vi "Save File Parse File Name.vi"(0 "File String Name":path, 1 "Number of Cycles/ File":i32=1, 5 "Error In":errorcluster, 6 "Initialize.Washer In":T1={"Appliance Details"={"FileVersionInfo"={"FileVersion"="", "ProductName"="", "InternalName"="", "CompanyName"="", "LegalCopyright"="", "FileDescription"=""}, "Dishwasher Info"={"Open Cup Weight (gm):"=0.0, "Auto Cup Weight (gm):"=0.0, "Detergent-Dish:"="", "Inlet Temperature-Dish:"="", "Cycle Mode-Dish:"="", "Unit Control-Dish:"="", "Manufacturer-Dish:"=""}, "Washer Info"={"Hot Water Temperature (Fahrenheit):"="", "Cold Water Temperature (Fahrenheit):"="", "Capacity (cu.ft):"=0.0, "Initial Cloth Weight:"=0.0, "Cloth Lot:"=0, "Model Family:"="", "Program Name:"="", "Cycle Selection:"="", "Wash Temperature:"="", "Rinse Temperature:"="", "Load Size:"=""}, "File Name Output Array"=[], "Calibration Output Array"=[], "Appliance Common"={"Engineer:"="", "Model Number:"="", "Serial Number:"="", "Comments:"="", "Station ID:"="", "Technician:"="", "TR Number:"="", "Lab ID:"="", "Voltage:"="", "Water Pressure (PSI):"="", "Test Date:"="", "Computer Name:"="", "IP Address:"="", "Ambient RH:"="", "Frequency:"="", "Build:"="", "Filename:"="", "Test Type:"="", "Load Run #:"=0, "Ambient Temperature (F):"="", "File Path:"=path "", "Cycles Per Year"=60}, "Water Heater"={"Heating Mode:"=""}, "Dryer"={"Heat Setting:"="", "Washer Water Temperature (60 ± 5°F):"=60, "Water Hardness (PPM):"=17, "Dryness Setting:"="", "Dryer Type:"="", "Exhaust:"="", "Drying Cycle:"="", "Load Type:"="", "Nominal Load Weight"="", "Dryer Initial IMC Data"={"Measured IMC (lbs)"=7.0, "Actual Initial RMC (%)"=7.0, "RMC (Desired %)"=100.0, "Bone Dry Wt(lbs)"=7.0, "Tolerance(%)"=5.0, "Actual Final RMC (%)"=0.0, "CEF (lbf/kWh)"=0.0, "Minimum Weight (lbf)"=0.0, "Average Weight (lbf)"=0.0, "Maximum Weight (lbf)"=0.0, "Measured IMC In Range?"=FALSE, "Moisture Reduction Factor"=55.5, "Field Use Factor"=1.04, "Empty Dryer Cold Weigth"=0.0, "Energy Standard"=enum."D2-Automatic Dryer", "Weight Cloth (lbs)"=0.0, "Relative Moisture Content (%)"=0.0, "Relative Moisture Content - Avg (%)"=0.0}}}, "Display Data (RLT)"={"Status Color"=0, "Serial Number Display"="", "Cycle Count Display"=0, "Station Label Display"="", "Current Run Start Time Display"=0.0, "Board ID Display"="", "RPM Display"=0, "Current Display"=0.0, "Current Path Display"=path "", "Saving Display"=FALSE, "Unit Type Display"=enum."", "Total Time On Display"=0.0, "UI Button"=FALSE}} {"Display Data (RLT)"."Current Display" format="%.2f"; "Display Data (RLT)"."Cycle Count Display" format="%04d"; "Appliance Details"."Dryer"."Dryer Initial IMC Data"."Maximum Weight (lbf)" format="%03_6g"; "Appliance Details"."Dryer"."Dryer Initial IMC Data"."Average Weight (lbf)" format="%03_6g"; "Appliance Details"."Dryer"."Dryer Initial IMC Data"."Minimum Weight (lbf)" format="%03_6g"; "Appliance Details"."Dryer"."Dryer Initial IMC Data"."CEF (lbf/kWh)" format="%03_6g"; "Appliance Details"."Dryer"."Dryer Initial IMC Data"."Actual Final RMC (%)" format="%03_6g"; "Appliance Details"."Dryer"."Dryer Initial IMC Data"."Tolerance(%)" format="%0#_6g"; "Appliance Details"."Dryer"."Dryer Initial IMC Data"."Bone Dry Wt(lbs)" format="%03_6g"; "Appliance Details"."Dryer"."Dryer Initial IMC Data"."RMC (Desired %)" format="%0#_6g"; "Appliance Details"."Dryer"."Dryer Initial IMC Data"."Actual Initial RMC (%)" format="%03_6g"; "Appliance Details"."Dryer"."Dryer Initial IMC Data"."Measured IMC (lbs)" format="%0#_6g"}) -> (14 "Root Change?":bool, 15 "New File?":bool, 19 "Error Out":errorcluster)   [LabVIEW 2023, in "Save File.lvlib"]
uses:
  Save File.lvlib
  Public/Type Definitions/Save File Washer.ctl
  File Setup (Public)/Type Definition/Save File DISH Dishwasher Details.ctl
  <vilib>/Platform/fileVersionInfo.llb/FileVersionInformation.ctl
  Washer DOE/Type Definitions/DOE Appliance Common.ctl
  Custom Pallet Controls/Custom Pallet String.ctl
  File Setup (Public)/Type Definition/DPT IMC Data.ctl
  Washer DOE/Type Definitions/DOE Dryer Standard.ctl
  Public/Type Definitions/Save File Appliance Display.ctl
  Public/Type Definitions/Save File Unit Type.ctl
  File Setup.lvlib
panel:
  in  "Appliance Details.Appliance Common.TR Number:":string
  in  "Appliance Details.Appliance Common.Lab ID:":string
  in  "Appliance Details.Appliance Common.Serial Number:":string
  in  "Display Data (RLT).Cycle Count Display":i32
  in  "Debug":bool
  out "Save Array":bool[](array[boolean])
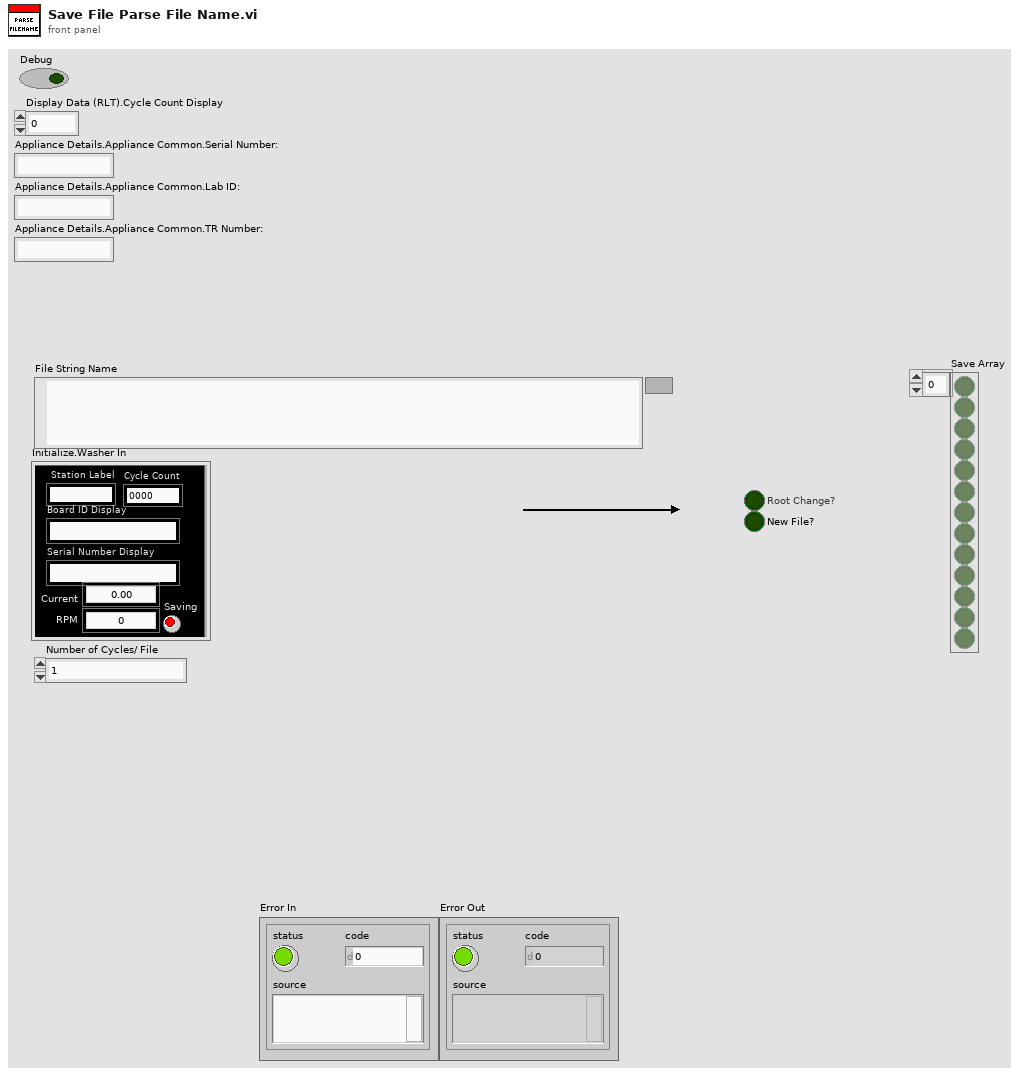
[diagram p1: front panel]
types:
  T1 = typedef "Save File.lvlib/Save File Washer.ctl" = cluster{"Appliance Details":T2, "Display Data (RLT)":T8}
  T2 = typedef "File Setup.lvlib/Save File DISH Dishwasher Details.ctl" = cluster{"FileVersionInfo":T3, "Dishwasher Info":cluster{"Open Cup Weight (gm):":dbl, "Auto Cup Weight (gm):":dbl, "Detergent-Dish:":string, "Inlet Temperature-Dish:":string, "Cycle Mode-Dish:":string, "Unit Control-Dish:":string, "Manufacturer-Dish:":string}, "Washer Info":cluster{"Hot Water Temperature (Fahrenheit):":string, "Cold Water Temperature (Fahrenheit):":string, "Capacity (cu.ft):":dbl, "Initial Cloth Weight:":dbl, "Cloth Lot:":i32, "Model Family:":string, "Program Name:":string, "Cycle Selection:":string, "Wash Temperature:":string, "Rinse Temperature:":string, "Load Size:":string}, "File Name Output Array":string[][], "Calibration Output Array":string[][], "Appliance Common":T4, "Water Heater":cluster{"Heating Mode:":string}, "Dryer":cluster{"Heat Setting:":T5, "Washer Water Temperature (60 ± 5°F):":u16, "Water Hardness (PPM):":u16, "Dryness Setting:":T5, "Dryer Type:":string, "Exhaust:":string, "Drying Cycle:":string, "Load Type:":string, "Nominal Load Weight":string, "Dryer Initial IMC Data":T6}}
  T3 = typedef "FileVersionInformation.ctl" = cluster{"FileVersion":string, "ProductName":string, "InternalName":string, "CompanyName":string, "LegalCopyright":string, "FileDescription":string}
  T4 = typedef "DOE Appliance Common.ctl" = cluster{"Engineer:":string, "Model Number:":string, "Serial Number:":string, "Comments:":string, "Station ID:":string, "Technician:":string, "TR Number:":string, "Lab ID:":string, "Voltage:":string, "Water Pressure (PSI):":string, "Test Date:":string, "Computer Name:":string, "IP Address:":string, "Ambient RH:":string, "Frequency:":string, "Build:":string, "Filename:":string, "Test Type:":string, "Load Run #:":i32, "Ambient Temperature (F):":string, "File Path:":path, "Cycles Per Year":u32}
  T5 = typedef "Custom Pallet String.ctl" = string
  T6 = typedef "DPT IMC Data.ctl" = cluster{"Measured IMC (lbs)":dbl, "Actual Initial RMC (%)":dbl, "RMC (Desired %)":dbl, "Bone Dry Wt(lbs)":dbl, "Tolerance(%)":dbl, "Actual Final RMC (%)":dbl, "CEF (lbf/kWh)":dbl, "Minimum Weight (lbf)":dbl, "Average Weight (lbf)":dbl, "Maximum Weight (lbf)":dbl, "Measured IMC In Range?":bool, "Moisture Reduction Factor":dbl, "Field Use Factor":dbl, "Empty Dryer Cold Weigth":dbl, "Energy Standard":T7, "Weight Cloth (lbs)":dbl, "Relative Moisture Content (%)":dbl, "Relative Moisture Content - Avg (%)":dbl}
  T7 = typedef "DOE Dryer Standard.ctl" = enum16{"D2-Automatic Dryer", "D2-Timer Dryer", "D1-Automatic Dryer", "D1-Timer Dryer", "Other"}
  T8 = typedef "Save File Appliance Display.ctl" = cluster{"Status Color":u32, "Serial Number Display":string, "Cycle Count Display":i32, "Station Label Display":string, "Current Run Start Time Display":dbl, "Board ID Display":string, "RPM Display":u32, "Current Display":dbl, "Current Path Display":path, "Saving Display":bool, "Unit Type Display":T9, "Total Time On Display":dbl, "UI Button":bool}
  T9 = typedef "Save File.lvlib/Save File Unit Type.ctl" = enum32{"", "Viper", "Hawk", "2015"}
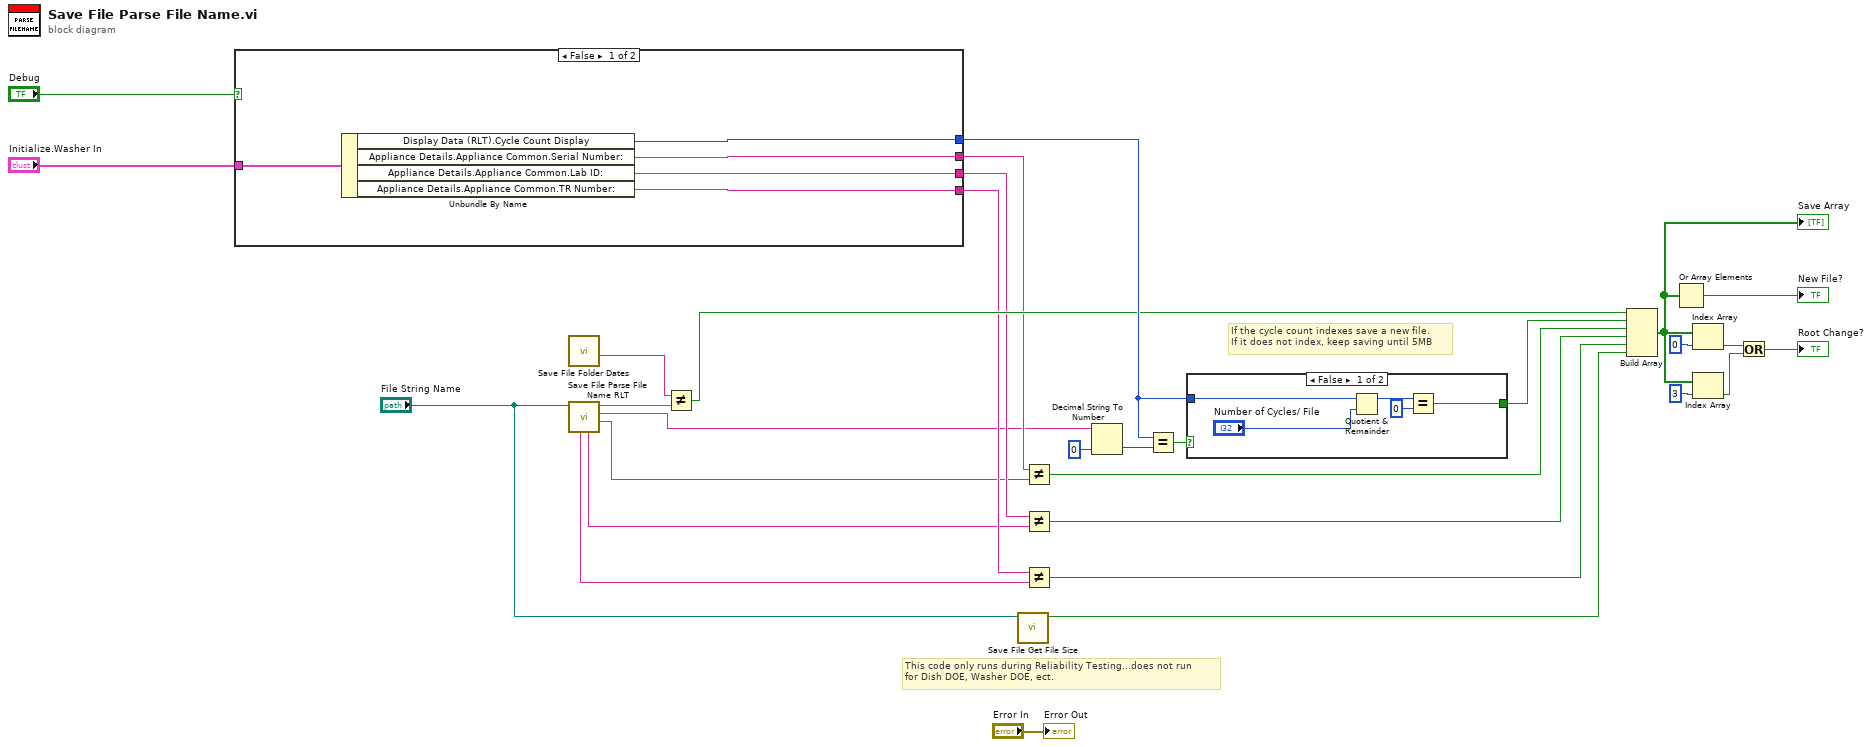
[diagram p0: block diagram]
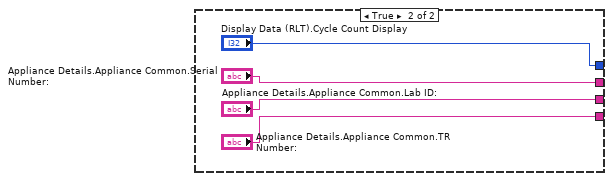
[diagram p2: hidden frame]
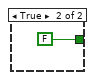
[diagram p3: hidden frame]
diagram:
  # "This code only runs during Reliability Testing...does not run \nfor Dish DOE, Washer DOE, ect."
  # "If the cycle count indexes save a new file.\nIf it does not index, keep saving until 5MB"
  n1 = case shown="False" "Debug" {
    tunnel: [w35 "Display Data (RLT).Cycle Count Display"] -> w27
    tunnel: "Initialize.Washer In" -> [w34 _]
    tunnel: [w33 "Appliance Details.Appliance Common.Serial Number:"] -> w11
    tunnel: [w32 "Appliance Details.Appliance Common.Lab ID:"] -> w10
    tunnel: [w31 "Appliance Details.Appliance Common.TR Number:"] -> w9
    frame False {
      n2 = Unbundle By Name(w34) -> ("Display Data (RLT).Cycle Count Display"=w35:i32, "Appliance Details.Appliance Common.Serial Number:"=w33:string, "Appliance Details.Appliance Common.Lab ID:"=w32:string, "Appliance Details.Appliance Common.TR Number:"=w31:string)
    }
    frame True {
    }
  }
  n3 = call "Save File Folder Dates.vi"() -> ("Year/Month/Day"=w28:string)  [unwired: 8 in, 3 out]
  n4 = call "Save File Parse File Name RLT.vi"("File String Name"="File String Name") -> ("Serial Number"=w3:string, "Cycle"=w4:string, "Date"=w7:string, "Lab ID"=w2:string, "TR Number"=w1:string)  [unwired: 5 in, 1 out]
  n5 = Not Equal?(x=w28, y=w7) -> (x != y?=w17:bool)
  n6 = call "Save File Get File Size.vi"("Old path"="File String Name") -> ("File Size Greater Than Limit"=w14:bool)  [unwired: 8 in, 2 out]
  n7 = Not Equal?(x=w11, y=w3) -> (x != y?=w13:bool)
  n8 = Not Equal?(x=w10, y=w2) -> (x != y?=w5:bool)
  n9 = Not Equal?(x=w9, y=w1) -> (x != y?=w12:bool)
  n10 = Decimal String To Number(string=w4, default (0L)=u16 0 ("default (0 I32)")) -> (number=w16:u16)  [unwired: 1 in, 1 out]
  n11 = Equal?(x=w27, y=w16) -> (x = y?=w25:bool)
  n12 = case shown="False" w25 {
    tunnel: w27 -> [w41 _]
    tunnel: [w40 FALSE] -> w26
    frame False {
      n13 = Quotient & Remainder(x=w41, y="Number of Cycles/ File") -> (x-y*floor(x/y)=w43:i32)  [unwired: 1 out]
      n14 = Equal?(x=w43, y=0) -> (x = y?=w40:bool)
    }
    frame True {
    }
  }
  n15 = Build Array(w17, w26, w13, w5, w12, w14) -> (w23:bool[])
  "Save Array" <- w23
  n16 = Or Array Elements(Boolean array=w23) -> (logical OR=→"New File?":bool)
  n17 = Index Array(array=w23, index=0) -> (element=w20:bool)
  n18 = Index Array(array=w23, index=3) -> (element=w19:bool)
  n19 = Or(x=w20, y=w19) -> (x .or. y?=→"Root Change?":bool)
  "Error Out" <- "Error In"
